vi "Wait to resume.vi"(5 "Auto close (s)":u32=120, 10 "Caption.Text":string) -> ()   [LabVIEW 2018]
panel:
  out "Windows close (s)":u32 caption="Window closes in"
  in  "Done":bool
  # "s"
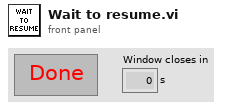
[diagram p1: front panel]
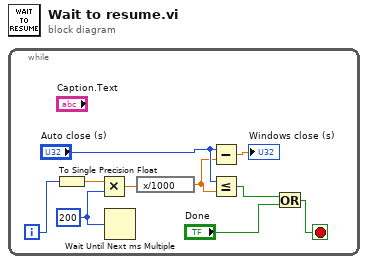
[diagram p0: block diagram]
diagram:
  n1 = while {
    i -> [w9]
    stop <- w7 stop-if-true
    w10 = u32 200 ("millisecond multiple")
    n2 = To Single Precision Float(number=w9) -> (single precision float=w1:sgl)
    n3 = Multiply(x=w1, y=w10) -> (x*y=w6:sgl)
    n4 = Wait Until Next ms Multiple(millisecond multiple=w10) -> ()  [unwired: 1 out]
    n5 = expression code="x/1000"(w6) -> (w3:sgl)
    n6 = Subtract(x="Auto close (s)", y=w3) -> (x-y=→"Windows close (s)":sgl)
    n7 = Less Or Equal?(x="Auto close (s)", y=w3) -> (x <= y?=w2:bool)
    n8 = Or(x=w2, y="Done") -> (x .or. y?=w7:bool)
  }
